vi "gen_coherent_sine.vi"(2 "fs [Hz]":dbl=48000.0, 3 "limit wave size to power of 2":bool, 4 "f in [Hz]":dbl=1000.0) -> (0 "wave":dbl[](array[numeric]), 1 "f out [Hz]":dbl=1000.0)   [LabVIEW 2013, in "dsdll.lvlib"]
doc: "This VI generates single sine wave period for given frequency and sampling rate. Nearest possible frequency is chosen to ensure periodic waveform."
uses:
  dsdll.lvlib
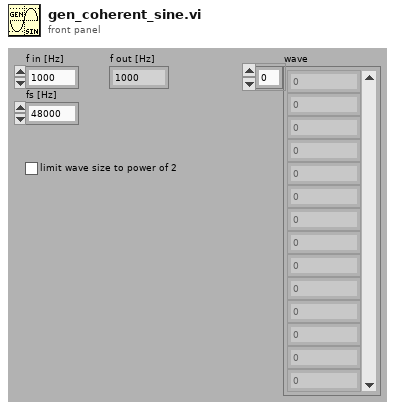
[diagram p1: front panel]
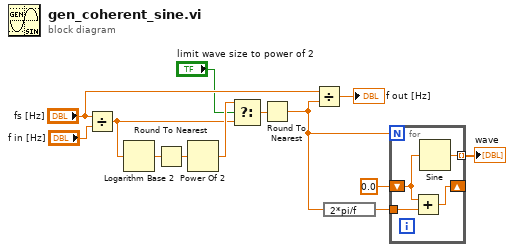
[diagram p0: block diagram]
diagram:
  n1 = Divide(x="fs [Hz]", y="f in [Hz]") -> (x/y=w4:dbl)
  n2 = Logarithm Base 2(1:w4) -> (0:w7:dbl)
  n3 = Round To Nearest(number=w7) -> (nearest integer value=w6:dbl)
  n4 = Power Of 2(x=w6) -> (2^x=w5:dbl)
  n5 = Select(t=w5, s="limit wave size to power of 2", f=w4) -> (s? t:f=w3:dbl)
  n6 = Round To Nearest(number=w3) -> (nearest integer value=w2:dbl)
  n7 = Divide(x="fs [Hz]", y=w2) -> (x/y=→"f out [Hz]":dbl)
  n8 = expression code="2*pi/f"(w2) -> (w9:dbl)
  n9 = for {
    N: w2 -> [_]
    shift-right: [w16] -> _
    shift-left: 0.0 -> [w15]
    tunnel: w9 -> [w17]
    tunnel: [w14] -> w8 mode=indexing
    n10 = Add(x=w15, y=w17) -> (x+y=w16:dbl)
    n11 = Sine(x=w15) -> (sin(x)=w14:dbl)
  }
  "wave" <- w8
